vi "Framework Host Sobot.vi"() -> ()   [LabVIEW 2017]
uses:
  TypeDefinitions/TCP Cluster.ctl
  TypeDefinitions/TCP Commands.ctl
  TypeDefinitions/Events.ctl
  <vilib>/Utility/inputDevices.llb/closeJoystick.vi
panel:
  out "Receive":T1={"Datatype"=enum."Message", "String"="Send to sobot"}
  in  "Device Index":i32
  in  "Manual Drive":bool
  out "Send":T1={"Datatype"=enum."Message", "String"="Send to sobot"}
  in  "Button 2":bool
  in  "Stop":bool
  in  "Button 1":bool
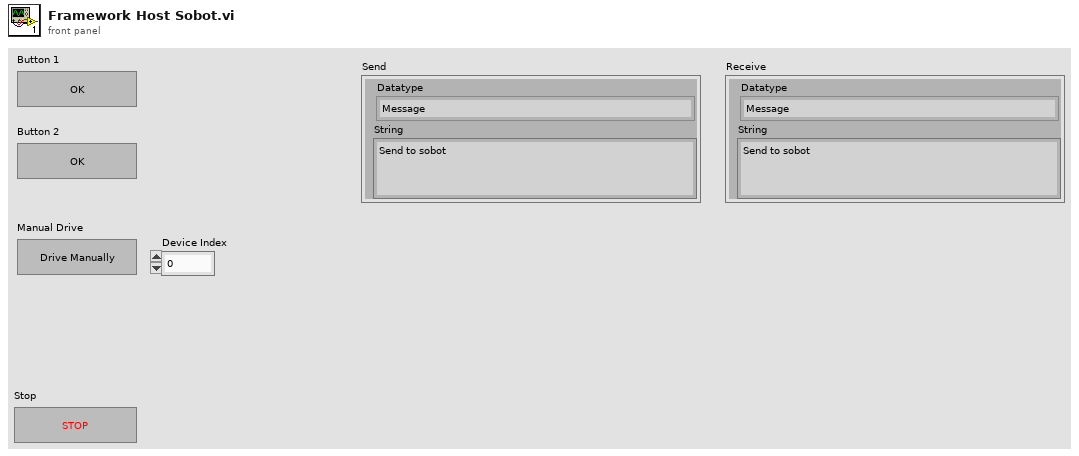
[diagram p1: front panel]
types:
  T1 = typedef "TCP Cluster.ctl" = cluster{"Datatype":T2, "String":string}
  T2 = typedef "TCP Commands.ctl" = enum16{"Timeout", "Log", "Message", "ManualDrive", "Stop", "Command"}
  T3 = typedef "Events.ctl" = enum16{"Timeout", "Stop", "Button 1", "Button 2", "StartManualDrive", "ManualDrive", "StopManualDrive"}
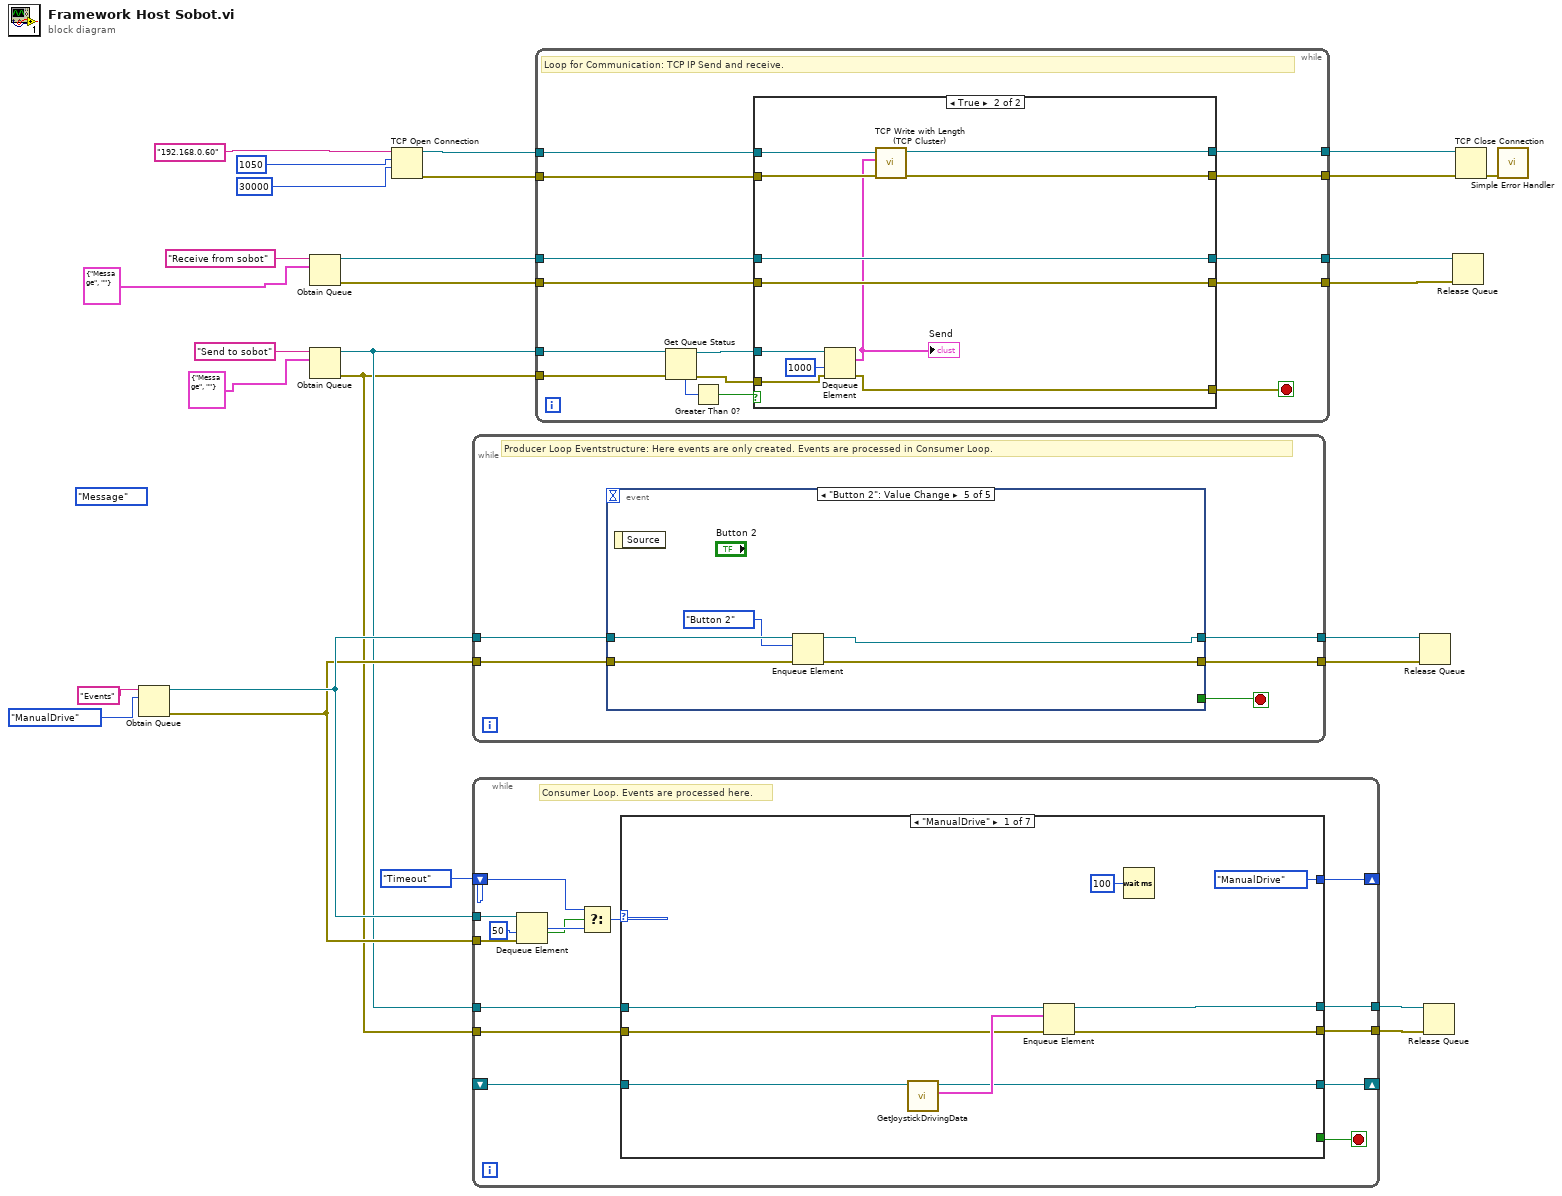
[diagram p0: block diagram]
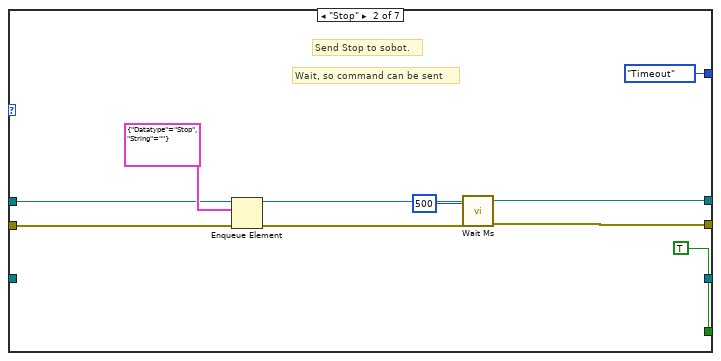
[diagram p2: hidden frame]
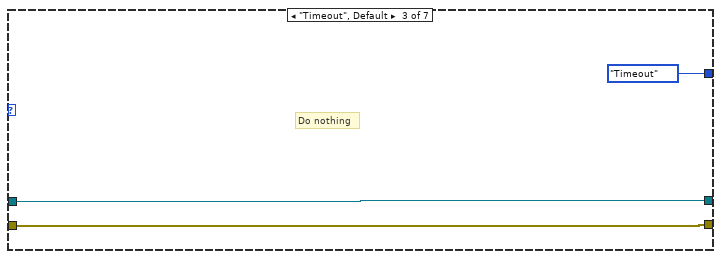
[diagram p3: hidden frame]
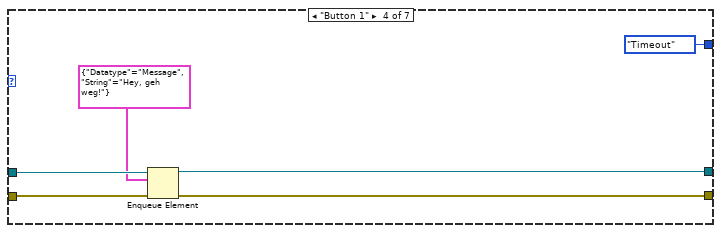
[diagram p4: hidden frame]
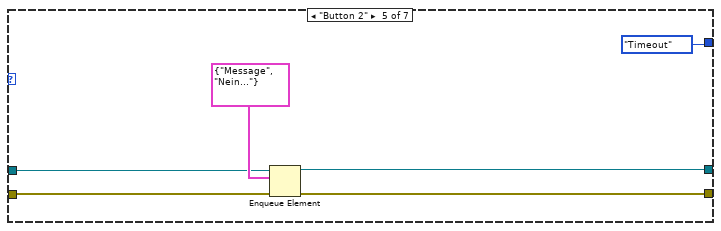
[diagram p5: hidden frame]
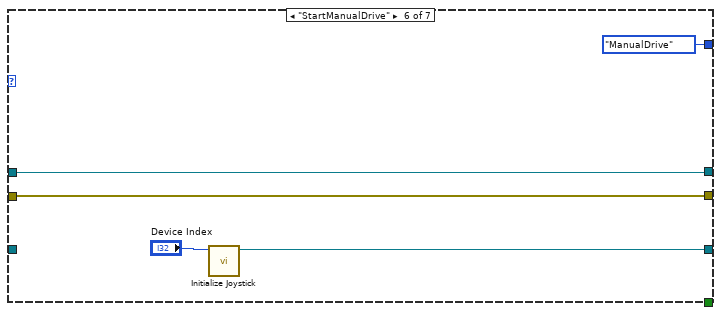
[diagram p6: hidden frame]
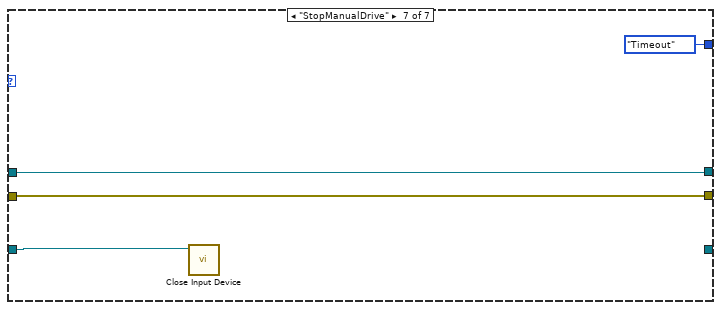
[diagram p7: hidden frame]
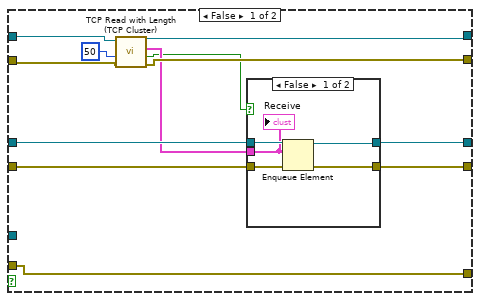
[diagram p8: hidden frame]
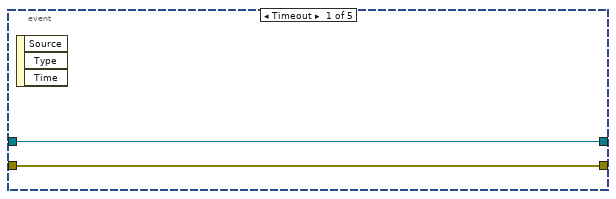
[diagram p10: hidden frame]
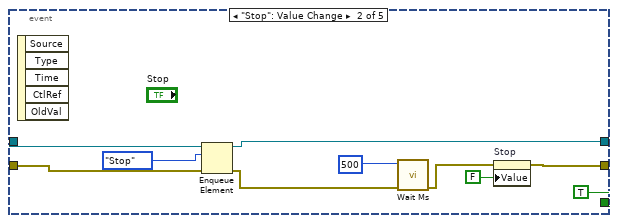
[diagram p11: hidden frame]
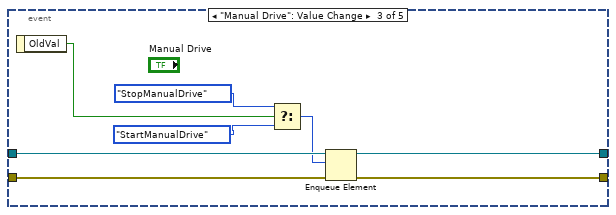
[diagram p12: hidden frame]
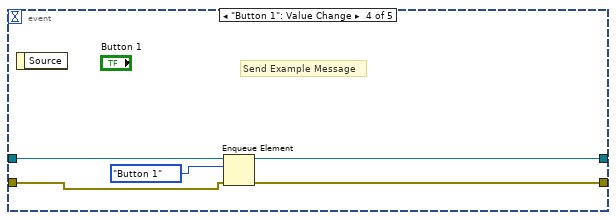
[diagram p13: hidden frame]
diagram:
  (unwired) TCP_Commands."Message"
  n1 = Obtain Queue(name (unnamed)="Events", element data type=Events."ManualDrive" ("Events")) -> (queue out=w7:refnum<queue>, error out=w6:errorcluster)  [unwired: 3 in, 1 out]
  n2 = Obtain Queue(name (unnamed)="Receive from sobot", element data type=T1 {"Datatype"=enum."Message", "String"=""}) -> (queue out=w22:refnum<queue>, error out=w21:errorcluster)  [unwired: 3 in, 1 out]
  n3 = Obtain Queue(name (unnamed)="Send to sobot", element data type=T1 {"Datatype"=enum."Message", "String"=""}) -> (queue out=w4:refnum<queue>, error out=w1:errorcluster)  [unwired: 3 in, 1 out]
  n4 = TCP Open Connection(address="192.168.0.60", remote port or service name=u16 1050, timeout ms (60000)=30000) -> (connection ID=w16:refnum<k5>, error out=w15:errorcluster)  [unwired: 2 in]
  n5 = while {
    tunnel: w7 -> [w31]
    tunnel: w6 -> [w30]
    tunnel: [w29] -> w9
    tunnel: [w28] -> w8
    stop <- w32 stop-if-true
    # "Producer Loop Eventstructure: Here events are only created. Events are processed in Consumer Loop."
    n6 = event shown="[4] \"Button 2\": Value Change" {
      selector: _ -> [_ _ _ _ _]
      dyn-events: _ -> [_ _ _ _ _]
      timeout: _ -> [_ _ _ _ _]
      tunnel: [_ TRUE _ _ _] -> w32
      tunnel: w31 -> [w34 w43 w52 w55 w62]
      tunnel: w30 -> [w33 w41 w51 w56 w61]
      tunnel: [w34 w35 w50 w54 w60] -> w29
      tunnel: [w33 w36 w49 w53 w59] -> w28
      event Timeout {
        n7 = event-data() -> ()  [unwired: 1 in, 3 out]
      }
      event "Stop": Value Change {
        n8 = event-data() -> ()  [unwired: 1 in, 5 out]
        n9 = Enqueue Element(queue=w43, element=Events."Stop" ("Events"), error in (no error)=w41) -> (queue out=w35:refnum<queue>, error out=w39:errorcluster)  [unwired: 1 in, 1 out]
        n10 = call "Wait Ms.vi"("error in (no error)"=w39, "milliseconds to wait"=u32 500) -> ("error out"=w37:errorcluster)  [unwired: 9 in]
        n11 = property on="Stop" class="Bool (strict)"(error in=w37, "Value"=FALSE ("stop")) -> (error out=w36:errorcluster)  [unwired: 1 in, 1 out]
      }
      event "Manual Drive": Value Change {
        n12 = event-data() -> ("OldVal"=w48:bool)  [unwired: 1 in]
        n13 = Select(t=Events."StopManualDrive" ("Events"), s=w48, f=Events."StartManualDrive" ("Events")) -> (s? t:f=w46:T3)
        n14 = Enqueue Element(queue=w52, element=w46, error in (no error)=w51) -> (queue out=w50:refnum<queue>, error out=w49:errorcluster)  [unwired: 1 in, 1 out]
      }
      event "Button 1": Value Change {
        # "Send Example Message"
        n15 = event-data() -> ()  [unwired: 1 in, 1 out]
        n16 = Enqueue Element(queue=w55, element=Events."Button 1" ("Events"), error in (no error)=w56) -> (queue out=w54:refnum<queue>, error out=w53:errorcluster)  [unwired: 1 in, 1 out]
      }
      event "Button 2": Value Change {
        n17 = event-data() -> ()  [unwired: 1 in, 1 out]
        n18 = Enqueue Element(queue=w62, element=Events."Button 2" ("Events"), error in (no error)=w61) -> (queue out=w60:refnum<queue>, error out=w59:errorcluster)  [unwired: 1 in, 1 out]
      }
    }
  }
  n19 = while {
    tunnel: w7 -> [w77]
    tunnel: w6 -> [w76]
    shift-right: [w73] -> _
    shift-left: Events."Timeout" ("Events") -> [w72]
    tunnel: w4 -> [w68]
    tunnel: [w67] -> w3
    tunnel: [w66] -> w2
    tunnel: w1 -> [w65]
    shift-right: [w64] -> _
    shift-left: _ -> [w63]
    stop <- w74 stop-if-true
    # "Consumer Loop. Events are processed here."
    n20 = Dequeue Element(queue=w77, timeout in ms (-1)=50, error in (no error)=w76) -> (element=w71:T3, timed out?=w69:bool)  [unwired: 2 out]
    n21 = Select(t=w72, s=w69, f=w71) -> (s? t:f=w70:T3)
    n22 = case shown="\"ManualDrive\"" w70 {
      tunnel: [_ TRUE _ _ _ _ _] -> w74
      tunnel: [Events."ManualDrive" ("Events") Events."Timeout" ("Events") Events."Timeout" ("Events") Events."Timeout" ("Events") Events."Timeout" ("Events") Events."ManualDrive" ("Events") Events."Timeout" ("Events")] -> w73
      tunnel: w68 -> [w84 w92 w97 w104 w109 w115 w118]
      tunnel: [w83 w91 w97 w101 w107 w115 w118] -> w67
      tunnel: [w78 w88 w96 w100 w106 w114 w117] -> w66
      tunnel: w65 -> [w79 w87 w96 w103 w108 w114 w117]
      tunnel: [w82 _ _ _ _ w112 _] -> w64
      tunnel: w63 -> [w81 _ _ _ _ _ w119]
      frame "ManualDrive" {
        n23 = call "GetJoystickDrivingData.vi"("Refnum in"=w81) -> ("DriveData"=w86:T1, "Refnum out"=w82:refnum<k1>)  [unwired: 6 in, 3 out]
        n24 = Enqueue Element(queue=w84, element=w86, error in (no error)=w79) -> (queue out=w83:refnum<queue>, error out=w78:errorcluster)  [unwired: 1 in, 1 out]
        n25 = Wait (ms)(milliseconds to wait=u32 100) -> ()  [unwired: 1 out]
      }
      frame "Stop" {
        # "Wait, so command can be sent"
        # "Send Stop to sobot."
        n26 = Enqueue Element(queue=w92, element=T1 {"Datatype"=enum."Stop", "String"=""}, error in (no error)=w87) -> (queue out=w91:refnum<queue>, error out=w89:errorcluster)  [unwired: 1 in, 1 out]
        n27 = call "Wait Ms.vi"("error in (no error)"=w89, "milliseconds to wait"=u32 500) -> ("error out"=w88:errorcluster)  [unwired: 9 in]
      }
      frame "Timeout", Default {
        # "Do nothing"
      }
      frame "Button 1" {
        n28 = Enqueue Element(queue=w104, element=T1 {"Datatype"=enum."Message", "String"="Hey, geh weg!"}, error in (no error)=w103) -> (queue out=w101:refnum<queue>, error out=w100:errorcluster)  [unwired: 1 in, 1 out]
      }
      frame "Button 2" {
        n29 = Enqueue Element(queue=w109, element=T1 {"Datatype"=enum."Message", "String"="Nein..."}, error in (no error)=w108) -> (queue out=w107:refnum<queue>, error out=w106:errorcluster)  [unwired: 1 in, 1 out]
      }
      frame "StartManualDrive" {
        n30 = call <vilib>:"Initialize Joystick.vi"("device index"="Device Index") -> ("device ID"=w112:refnum<k1>)  [unwired: 9 in, 1 out]
      }
      frame "StopManualDrive" {
        n31 = call-poly <vilib>:"Close Input Device.vi"("device ID"=w119) -> ()  [unwired: 9 in, 1 out]
      }
    }
  }
  n32 = while {
    tunnel: w4 -> [w133]
    tunnel: w1 -> [w131]
    tunnel: w16 -> [w127]
    tunnel: w15 -> [w126]
    tunnel: [w125] -> w25
    tunnel: [w124] -> w24
    tunnel: w22 -> [w123]
    tunnel: w21 -> [w122]
    tunnel: [w121] -> w19
    tunnel: [w120] -> w20
    stop <- w134 stop-if-true
    # "Loop for Communication: TCP IP Send and receive."
    n33 = Get Queue Status(queue=w133, error in (no error)=w131) -> (queue out=w132:refnum<queue>, error out=w130:errorcluster, # elements in queue=w129:i32)  [unwired: 1 in, 5 out]
    n34 = Greater Than 0?(x=w129) -> (x > 0?=w128:bool)
    n35 = case shown="True" w128 {
      tunnel: [w146 w164] -> w134
      tunnel: w132 -> [_ w162]
      tunnel: w130 -> [w146 w161]
      tunnel: w127 -> [w141 w158]
      tunnel: w126 -> [w140 w157]
      tunnel: [w138 w156] -> w124
      tunnel: [w137 w155] -> w125
      tunnel: w123 -> [w145 w160]
      tunnel: w122 -> [w144 w159]
      tunnel: [w143 w160] -> w120
      tunnel: [w142 w159] -> w121
      frame False {
        n36 = call "TCP Read with Length (TCP Cluster).vi"("error in (no error)"=w140, "Timeout"=50, "connection ID"=w141) -> ("error out"=w138:errorcluster, "Timeout?"=w135:bool, "TCP Cluster"=w136:T1, "connection ID out"=w137:refnum<k5>)  [unwired: 5 in]
        n37 = case shown="False" w135 {
          tunnel: w145 -> [w151 w153]
          tunnel: w144 -> [w150 w152]
          tunnel: w136 -> [w149 _]
          tunnel: [w148 w153] -> w143
          tunnel: [w147 w152] -> w142
          frame False {
            n38 = Enqueue Element(queue=w151, element=w149, error in (no error)=w150) -> (queue out=w148:refnum<queue>, error out=w147:errorcluster)  [unwired: 1 in, 1 out]
            "Receive" <- w149
          }
          frame True {
          }
        }
      }
      frame True {
        n39 = Dequeue Element(queue=w162, timeout in ms (-1)=1000, error in (no error)=w161) -> (element=w154:T1, error out=w164:errorcluster)  [unwired: 2 out]
        "Send" <- w154
        n40 = call "TCP Write with Length (TCP Cluster).vi"("error in (no error)"=w157, 10:w154, "connection ID"=w158) -> ("error out"=w156:errorcluster, "connection ID out"=w155:refnum<k5>)  [unwired: 7 in]
      }
    }
  }
  n41 = Release Queue(queue=w9, error in (no error)=w8) -> ()  [unwired: 1 in, 3 out]
  n42 = Release Queue(queue=w3, error in (no error)=w2) -> ()  [unwired: 1 in, 3 out]
  n43 = Release Queue(queue=w20, error in (no error)=w19) -> ()  [unwired: 1 in, 3 out]
  n44 = TCP Close Connection(connection ID=w25, error in (no error)=w24) -> (error out=w26:errorcluster)  [unwired: 1 in, 1 out]
  n45 = call <vilib>:"Simple Error Handler.vi"("error in (no error)"=w26) -> ()  [unwired: 4 in, 5 out]
